vi "LVProjectShortcut_Item_NotifyChanged.vi"(8 "error in":errorcluster, 10 "Change Type":T1=enum."Item Modified", 11 "Object":T2) -> (0 "error out":errorcluster)   [LabVIEW 2017]
uses:
  <resource>/Framework/Providers/API/ItemRef.ctl
  <resource>/Framework/Providers/API/mxLvChangeType.ctl
  <resource>/Framework/Providers/API/mxLvUpdateUI.ctl
  <resource>/Framework/Providers/API/mxLvOverlayState.ctl
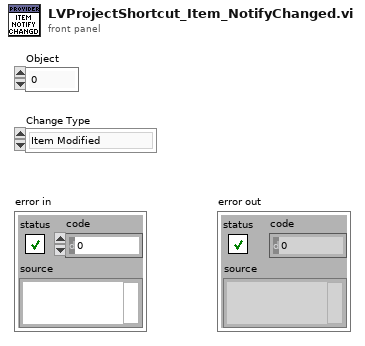
[diagram p1: front panel]
types:
  T1 = typedef "mxLvChangeType.ctl" = enum32{"Item Created", "Item Modified", "File Modified", "File Deleted", "Item Added", "Item Added to SCC", "Item Renamed", "Item Modified For SCC"}
  T2 = typedef "ItemRef.ctl" = u64
  T3 = typedef "mxLvUpdateUI.ctl" = cluster{"Action":u32, "Optional param 1":string, "Optional param 2":i32, "Optional param 3":string}
  T4 = typedef "mxLvOverlayState.ctl" = cluster{"Overlay Alias":string, "Active":bool}
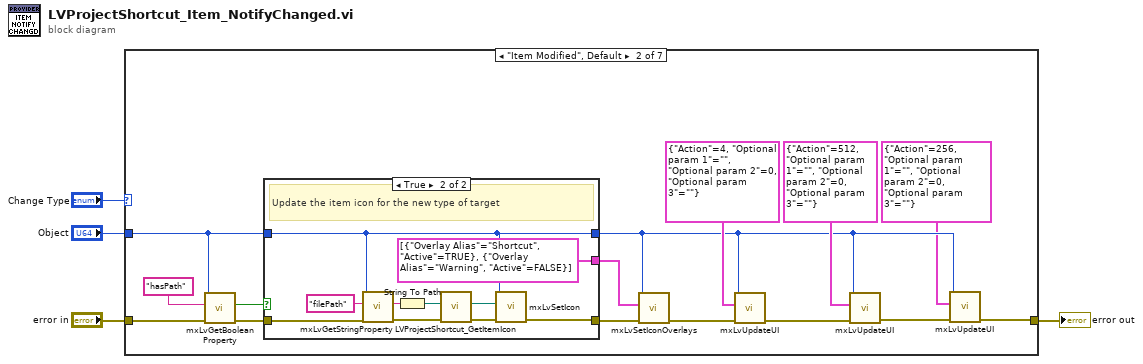
[diagram p0: block diagram]
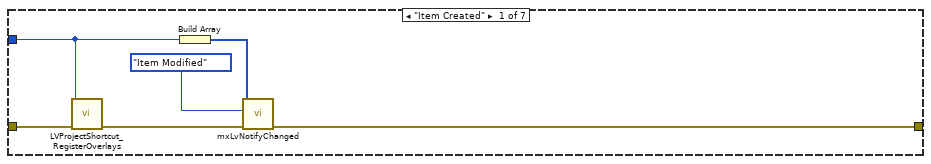
[diagram p2: hidden frame]
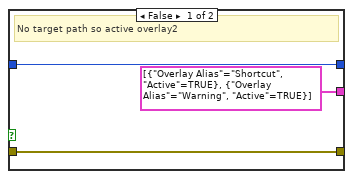
[diagram p3: hidden frame]
diagram:
  n1 = case shown="\"Item Modified\", Default" "Change Type" {
    tunnel: "error in" -> [w10 w24 w39 w40 w41 w42 w43]
    tunnel: "Object" -> [w7 w20 _ _ _ _ _]
    tunnel: [w5 w13 w39 w40 w41 w42 w43] -> w1
    frame "Item Created" {
      n2 = call "LVProjectShortcut_RegisterOverlays.vi"("error in"=w10, "Item"=w7) -> ("error out"=w6:errorcluster)  [unwired: 9 in]
      n3 = Build Array(w7) -> (w9:T2[])
      n4 = call <resource>:"mxLvNotifyChanged.vi"("error in (no error)"=w6, "Change Type"=mxLvChangeType."Item Modified", "Items"=w9) -> ("error out"=w5:errorcluster)  [unwired: 7 in, 1 out]
    }
    frame "Item Modified", Default {
      n5 = call <resource>:"mxLvGetBooleanProperty.vi"("error in"=w24, "Tag"="hasPath", "Item"=w20) -> ("error out"=w23:errorcluster, "Value"=w18:bool)  [unwired: 6 in, 1 out]
      n6 = case shown="True" w18 {
        tunnel: w23 -> [w28 w31]
        tunnel: [w28 w30] -> w21
        tunnel: w20 -> [w27 w29]
        tunnel: [w27 w29] -> w12
        tunnel: [T4[] [{"Overlay Alias"="Shortcut", "Active"=TRUE}, {"Overlay Alias"="Warning", "Active"=TRUE}] ("Overlay States") T4[] [{"Overlay Alias"="Shortcut", "Active"=TRUE}, {"Overlay Alias"="Warning", "Active"=FALSE}] ("Overlay States")] -> w17
        frame False {
          # "No target path so active overlay2"
        }
        frame True {
          # "Update the item icon for the new type of target"
          n7 = call <resource>:"mxLvGetStringProperty.vi"("Error In"=w31, "Tag"="filePath", "Item"=w29) -> ("Error Out"=w35:errorcluster, "Value"=w36:string)  [unwired: 6 in, 1 out]
          n8 = String To Path(string=w36) -> (path=w34:path)
          n9 = call "LVProjectShortcut_GetItemIcon.vi"("error in (no error)"=w35, "File Path"=w34) -> ("error out"=w32:errorcluster, "Icon Path"=w33:path)  [unwired: 8 in]
          n10 = call <resource>:"mxLvSetIcon.vi"("error in"=w32, "Icon Path"=w33, "Item"=w29) -> ("error out"=w30:errorcluster)  [unwired: 7 in, 1 out]
        }
      }
      n11 = call <resource>:"mxLvSetIconOverlays.vi"("error in"=w21, "Overlay States"=w17, "Item"=w12) -> ("error out"=w22:errorcluster)  [unwired: 7 in, 1 out]
      n12 = call <resource>:"mxLvUpdateUI.vi"("error in"=w22, "Update UI Settings"=T3 {"Action"=4, "Optional param 1"="", "Optional param 2"=0, "Optional param 3"=""}, "Item"=w12) -> ("error out"=w16:errorcluster)  [unwired: 7 in, 1 out]
      n13 = call <resource>:"mxLvUpdateUI.vi"("error in"=w16, "Update UI Settings"=T3 {"Action"=512, "Optional param 1"="", "Optional param 2"=0, "Optional param 3"=""}, "Item"=w12) -> ("error out"=w14:errorcluster)  [unwired: 7 in, 1 out]
      n14 = call <resource>:"mxLvUpdateUI.vi"("error in"=w14, "Update UI Settings"=T3 {"Action"=256, "Optional param 1"="", "Optional param 2"=0, "Optional param 3"=""}, "Item"=w12) -> ("error out"=w13:errorcluster)  [unwired: 7 in, 1 out]
    }
    frame "File Modified" {
    }
    frame "Item Added" {
    }
    frame "Item Added to SCC" {
    }
    frame "Item Renamed" {
    }
    frame "Item Modified For SCC" {
    }
  }
  "error out" <- w1
